vi "Z_State_heating.vi"(9 "Time":u32[](array[numeric])=[1000, 10000], 10 "Alarm":bool[](array[boolean])=[FALSE, FALSE], 11 "Z_In":T5={"Z_Source"=enum."local disabled", "Z_SetState"=enum."alarm", "ZM_State"=enum."initialization"}) -> (1 "t":u32, 3 "Z_Out":T4={"Z_Source"=enum."local disabled", "Z_State"=enum."alarm", "ZM_State"=enum."initialization"})   [LabVIEW 2019, in "Heating.lvlib"]
uses:
  Heating.lvlib
  ctl/Z_source.ctl
  ctl/Z_State.ctl
  ctl/ZM_State.ctl
  Trigers/RS.vi
  Timer Delay/Timer.vi
  Userlib.lvlib
panel:
  # "Alarm_L1"
  # "Alarm_L2"
  # "TsStop"
  # "T_check"
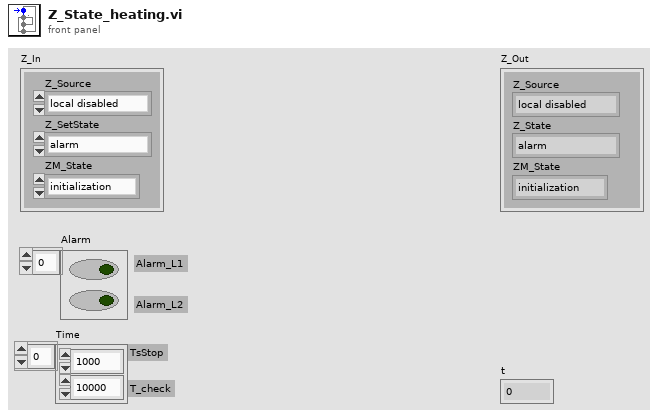
[diagram p1: front panel]
types:
  T1 = typedef "Heating.lvlib/Z_source.ctl" = enum8{"initialize", "local disabled", "local hand", "hand", "auto", "dist"}
  T2 = typedef "Heating.lvlib/Z_State.ctl" = enum8{"initialization", "alarm", "disabled", "not ready", "stop ready", "reserv", "switched off", "reserv2", "switched on", "check", "on min", "decrease out", "on", "increase out", "on max"}
  T3 = typedef "Heating.lvlib/ZM_State.ctl" = enum8{"initialization", "stop", "start_cmd", "contactor_on_cmd", "heating", "on", "stop_cmd", "power_down", "contactor_off_cmd", "cooling", "restart_delay"}
  T4 = cluster{"Z_Source":T1, "Z_State":T2, "ZM_State":T3}
  T5 = cluster{"Z_Source":T1, "Z_SetState":T2, "ZM_State":T3}
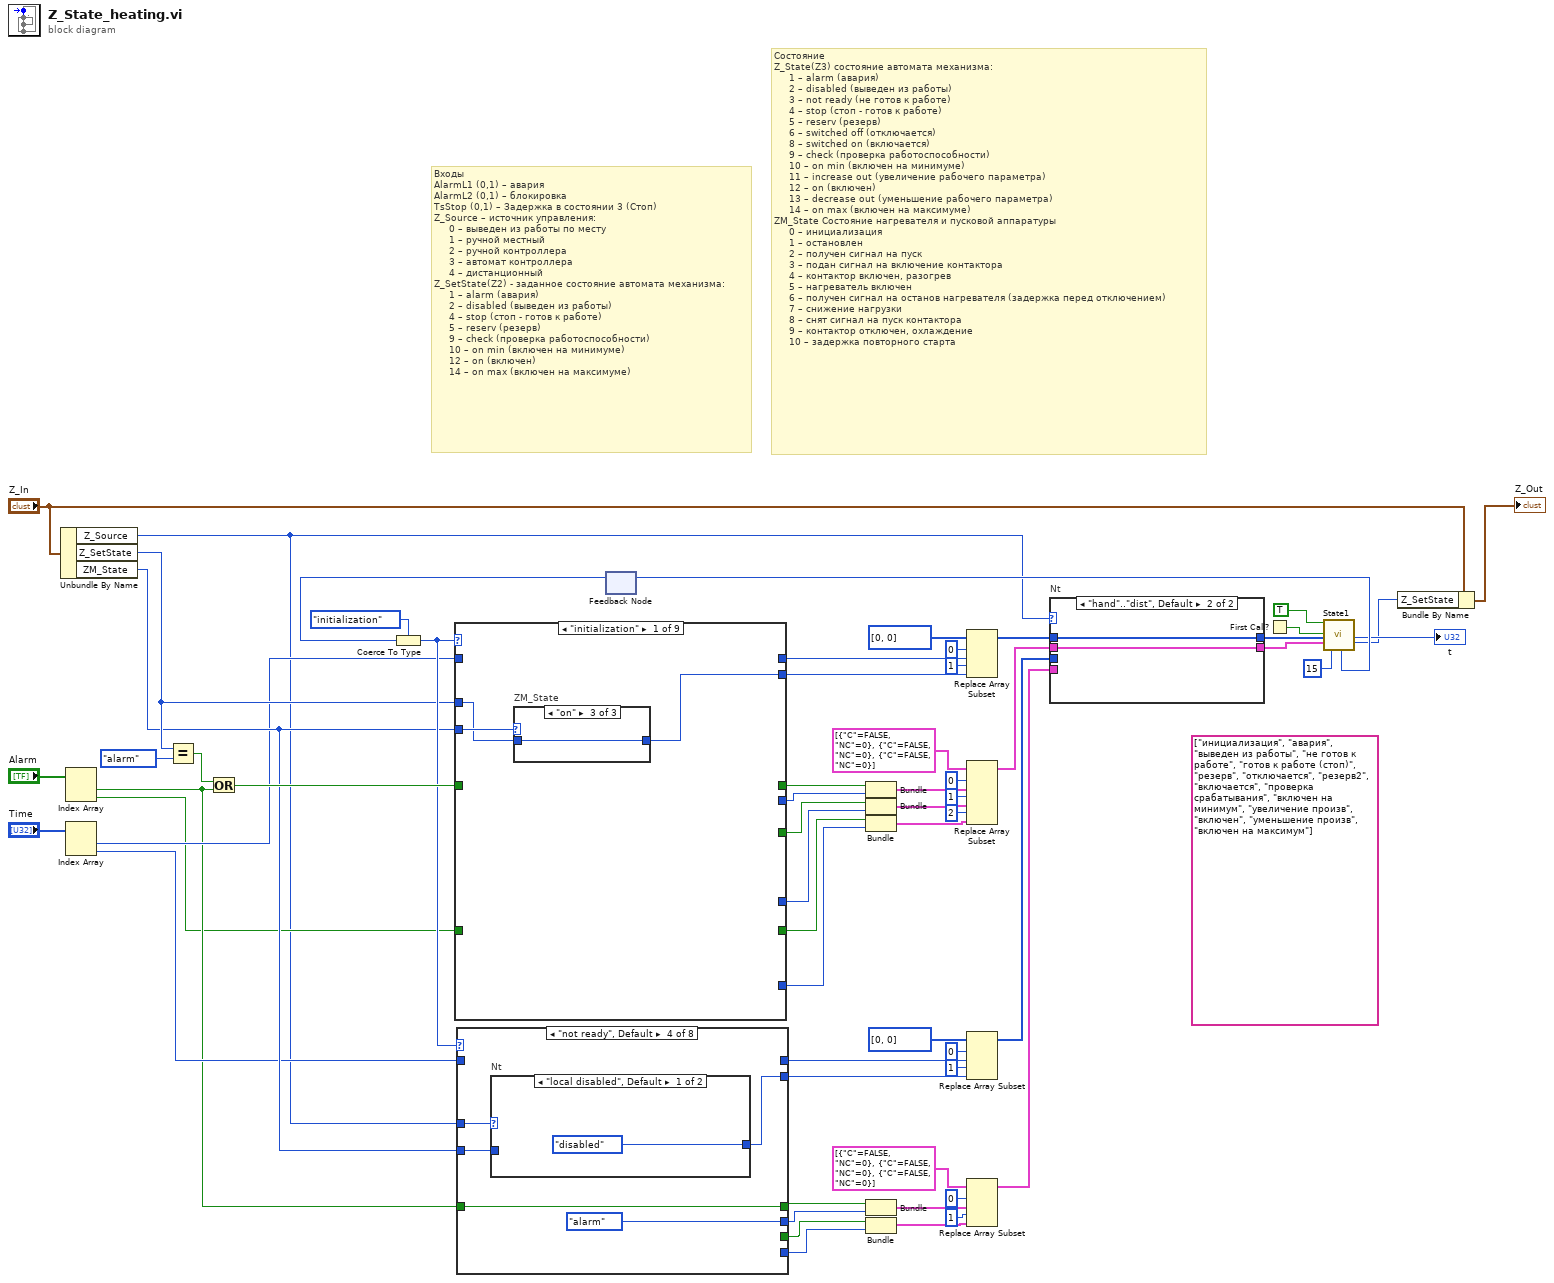
[diagram p0: block diagram]
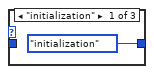
[diagram p3: hidden frame]
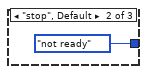
[diagram p4: hidden frame]
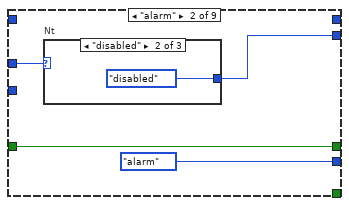
[diagram p5: hidden frame]
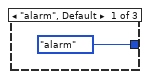
[diagram p6: hidden frame]
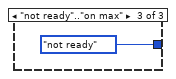
[diagram p7: hidden frame]
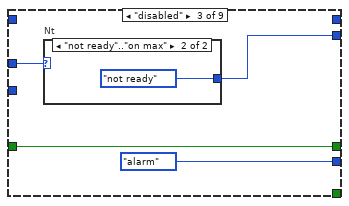
[diagram p8: hidden frame]
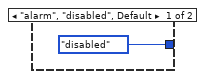
[diagram p9: hidden frame]
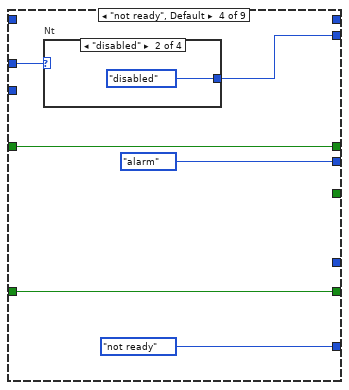
[diagram p10: hidden frame]
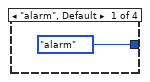
[diagram p11: hidden frame]
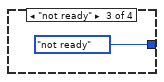
[diagram p12: hidden frame]
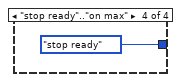
[diagram p13: hidden frame]
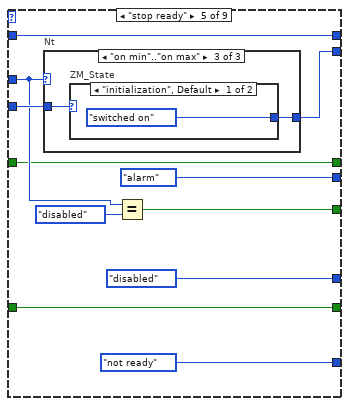
[diagram p14: hidden frame]
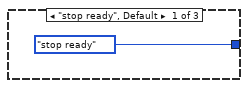
[diagram p15: hidden frame]
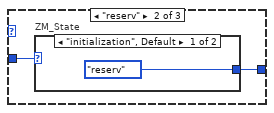
[diagram p16: hidden frame]
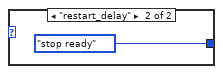
[diagram p17: hidden frame]
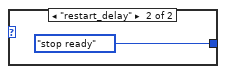
[diagram p18: hidden frame]
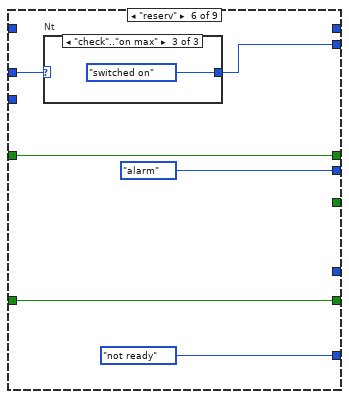
[diagram p19: hidden frame]
diagram:
  (unwired) string[] ["инициализация", "авария", "выведен из работы", "не готов к работе", "готов к работе (стоп)", "резерв", "отключается", "резерв2", "включается", "проверка срабатывания", "включен на минимум", "увеличение произв", "включен", "уменьшение произв", "включен на максимум"]
  # "Входы\nAlarmL1 (0,1) – авария\nAlarmL2 (0,1) – блокировка\nTsStop (0,1) – Задержка в состоянии 3 (Стоп)\nZ_Source – источник управления:\n     0 – выведен из работы по месту\n     1 – ручной местный\n     2 – ручной контроллера\n     3 – автомат контроллера\n     4 – дистанционный\nZ_SetState(Z2) - заданное состояние автомата механизма:\n     1 – alarm (авария)\n     2 – disabled (выведен из работы)\n     4 – stop (стоп - готов к работе)\n     5 – reserv (резерв)\n     9 – check (проверка работоспособности)\n     10 – on min (включен на минимуме)\n     12 – on (включен)\n     14 – on max (включен на максимуме)"
  # "Состояние\nZ_State(Z3) состояние автомата механизма:\n     1 – alarm (авария)\n     2 – disabled (выведен из работы)\n     3 – not ready (не готов к работе)\n     4 – stop (стоп - готов к работе)\n     5 – reserv (резерв)\n     6 – switched off (отключается)\n     8 – switched on (включается)\n     9 – check (проверка работоспособности)\n     10 – on min (включен на минимуме)\n     11 – increase out (увеличение рабочего параметра)\n     12 – on (включен)\n     13 – decrease out (уменьшение рабочего параметра)\n     14 – on max (включен на максимуме)\nZM_State Состояние нагревателя и пусковой аппаратуры\n     0 – инициализация\n     1 – остановлен\n     2 – получен сигнал на пуск\n     3 – подан сигнал на включение контактора\n     4 – контактор включен, разогрев\n     5 – нагреватель включен\n     6 – получен сигнал на останов нагревателя (задержка перед отключением)\n     7 – снижение нагрузки\n     8 – снят сигнал на пуск контактора\n     9 – контактор отключен, охлаждение\n     10 – задержка повторного старта"
  n1 = Unbundle By Name("Z_In") -> ("Z_Source"=w2:T1, "Z_SetState"=w55:T2, "ZM_State"=w54:T3)
  n2 = Index Array(array="Alarm") -> (element #1=w48:bool, element #2=w47:bool)  [unwired: 2 in]
  n3 = Index Array(array="Time") -> (element #1=w51:u32, element #2=w50:u32)  [unwired: 2 in]
  n4 = Equal?(x=w55, y=Z_State."alarm") -> (x = y?=w61:bool)
  n5 = Or(x=w61, y=w48) -> (x .or. y?=w60:bool)
  n6 = feedback #1() -> (w57:u32)  [unwired: 1 in]
  n7 = Coerce To Type(0:w57, 1:Z_State."initialization" ("Z_SetState")) -> (2:w56:T2)
  n8 = case shown="\"initialization\"" w56 {
    tunnel: w60 -> [_ w70 w77 w85 w95 w115 w127 w143 w158]
    tunnel: w55 -> [w62 w71 w78 w86 w99 w116 w128 w141 w154]
    tunnel: w47 -> [_ _ _ w83 w97 w114 w124 w144 w156]
    tunnel: w51 -> [_ _ _ _ w98 _ _ _ _]
    tunnel: w54 -> [w64 _ _ _ w100 _ w121 w147 _]
    tunnel: [_ _ _ Z_State."not ready" ("Z_SetState") Z_State."not ready" ("Z_SetState") Z_State."not ready" ("Z_SetState") w120 Z_State."switched off" ("Z_SetState") Z_State."switched off" ("Z_SetState")] -> w10
    tunnel: [_ _ _ _ w98 _ _ _ _] -> w16
    tunnel: [_ _ _ w83 w97 w114 w124 w146 w157] -> w9
    tunnel: [_ _ _ _ Z_State."disabled" ("Z_SetState") _ w125 _ _] -> w8
    tunnel: [_ _ _ _ w96 _ w126 _ _] -> w11
    tunnel: [_ Z_State."alarm" ("Z_SetState") Z_State."alarm" ("Z_SetState") Z_State."alarm" ("Z_SetState") Z_State."alarm" ("Z_SetState") Z_State."alarm" ("Z_SetState") Z_State."alarm" ("Z_SetState") Z_State."alarm" ("Z_SetState") Z_State."alarm" ("Z_SetState")] -> w12
    tunnel: [_ w70 w77 w85 w95 w115 w127 w143 w158] -> w13
    tunnel: [w63 w69 w76 w84 w94 w113 w123 w142 w154] -> w15
    frame "initialization" {
      n9 = case "ZM_State" shown="\"on\"" w64 {
        tunnel: [Z_State."initialization" ("Z_SetState") Z_State."not ready" ("Z_SetState") w67] -> w63
        tunnel: w62 -> [_ _ w67]
        frame "initialization" {
        }
        frame "stop", Default {
        }
        frame "on" {
        }
      }
    }
    frame "alarm" {
      n10 = case "Nt" shown="\"disabled\"" w71 {
        tunnel: [Z_State."alarm" ("Z_SetState") Z_State."disabled" ("Z_SetState") Z_State."not ready" ("Z_SetState")] -> w69
        frame "alarm", Default {
        }
        frame "disabled" {
        }
        frame "not ready".."on max" {
        }
      }
    }
    frame "disabled" {
      n11 = case "Nt" shown="\"not ready\"..\"on max\"" w78 {
        tunnel: [Z_State."disabled" ("Z_SetState") Z_State."not ready" ("Z_SetState")] -> w76
        frame "alarm", "disabled", Default {
        }
        frame "not ready".."on max" {
        }
      }
    }
    frame "not ready", Default {
      n12 = case "Nt" shown="\"disabled\"" w86 {
        tunnel: [Z_State."alarm" ("Z_SetState") Z_State."disabled" ("Z_SetState") Z_State."not ready" ("Z_SetState") Z_State."stop ready" ("Z_SetState")] -> w84
        frame "alarm", Default {
        }
        frame "disabled" {
        }
        frame "not ready" {
        }
        frame "stop ready".."on max" {
        }
      }
    }
    frame "stop ready" {
      n13 = case "Nt" shown="\"on min\"..\"on max\"" w99 {
        tunnel: [Z_State."stop ready" ("Z_SetState") w103 w107] -> w94
        tunnel: w100 -> [_ w104 w108]
        frame "stop ready", Default {
        }
        frame "reserv" {
          n14 = case "ZM_State" shown="\"initialization\", Default" w104 {
            tunnel: [Z_State."reserv" ("Z_SetState") Z_State."stop ready" ("Z_SetState")] -> w103
            frame "initialization", Default {
            }
            frame "restart_delay" {
            }
          }
        }
        frame "on min".."on max" {
          n15 = case "ZM_State" shown="\"initialization\", Default" w108 {
            tunnel: [Z_State."switched on" ("Z_SetState") Z_State."stop ready" ("Z_SetState")] -> w107
            frame "initialization", Default {
            }
            frame "restart_delay" {
            }
          }
        }
      }
      n16 = Equal?(x=w99, y=Z_State."disabled") -> (x = y?=w96:bool)
    }
    frame "reserv" {
      n17 = case "Nt" shown="\"check\"..\"on max\"" w116 {
        selector: w116 -> [w117 _ _]
        tunnel: [w117 Z_State."stop ready" ("Z_SetState") Z_State."switched on" ("Z_SetState")] -> w113
        frame "alarm".."not ready", "reserv" {
        }
        frame "stop ready", Default {
        }
        frame "check".."on max" {
        }
      }
    }
    frame "switched off" {
      n18 = case "Nt" shown="\"stop ready\", \"reserv\", \"check\", Default" w128 {
        tunnel: [w134 Z_State."switched on" ("Z_SetState")] -> w123
        tunnel: w121 -> [w135 _]
        frame "stop ready", "reserv", "check", Default {
          n19 = case "ZM_State" shown="\"initialization\", Default" w135 {
            tunnel: [Z_State."stop ready" ("Z_SetState") Z_State."switched off" ("Z_SetState")] -> w134
            frame "initialization", Default {
            }
            frame "stop_cmd".."cooling" {
            }
          }
        }
        frame "on min".."on max" {
        }
      }
      n20 = case "ZM_State" shown="\"stop_cmd\"..\"cooling\"" w121 {
        tunnel: [Z_State."disabled" ("Z_SetState") Z_State."switched off" ("Z_SetState")] -> w125
        frame "initialization", "stop", "restart_delay", Default {
        }
        frame "stop_cmd".."cooling" {
        }
      }
      n21 = case "ZM_State" shown="\"initialization\", \"stop\", \"restart_delay\", Default" w121 {
        tunnel: [Z_State."not ready" ("Z_SetState") Z_State."switched off" ("Z_SetState")] -> w120
        frame "initialization", "stop", "restart_delay", Default {
        }
        frame "stop_cmd".."cooling" {
        }
      }
      n22 = Equal?(x=w128, y=Z_State."disabled") -> (x = y?=w126:bool)
    }
    frame "switched on" {
      n23 = case "ZM_State" shown="\"on\"" w147 {
        tunnel: [Z_State."switched on" ("Z_SetState") w149] -> w142
        tunnel: w141 -> [_ w149]
        frame "initialization", Default {
        }
        frame "on" {
        }
      }
      n24 = case "Z2" shown="\"disabled\"..\"reserv\", Default" w141 {
        tunnel: [FALSE TRUE] -> w145
        frame "check".."on max" {
        }
        frame "disabled".."reserv", Default {
        }
      }
      n25 = Or(x=w145, y=w144) -> (x .or. y?=w146:bool)
    }
    frame "check".."on max" {
      n26 = case "Z2" shown="\"disabled\"..\"reserv\", Default" w154 {
        tunnel: [FALSE TRUE] -> w155
        frame "check".."on max" {
        }
        frame "disabled".."reserv", Default {
        }
      }
      n27 = Or(x=w155, y=w156) -> (x .or. y?=w157:bool)
    }
  }
  n28 = case shown="\"not ready\", Default" w56 {
    tunnel: w48 -> [_ w169 _ w180 w190 w200 w210 w220]
    tunnel: w2 -> [_ w168 w173 w179 w189 _ _ _]
    tunnel: w54 -> [w162 _ _ w177 w188 w199 w209 w218]
    tunnel: [_ _ _ _ _ _ w208 _] -> w3
    tunnel: [_ _ _ _ _ _ w207 _] -> w4
    tunnel: [_ Z_State."alarm" ("Z_SetState") _ Z_State."alarm" ("Z_SetState") Z_State."alarm" ("Z_SetState") Z_State."alarm" ("Z_SetState") Z_State."alarm" ("Z_SetState") Z_State."alarm" ("Z_SetState")] -> w5
    tunnel: [_ w169 _ w180 w190 w200 w210 w220] -> w6
    tunnel: [w161 w167 w172 w178 w187 w198 w208 w217] -> w7
    tunnel: w50 -> [_ _ _ _ _ _ w206 _]
    tunnel: [_ _ _ _ _ _ w206 _] -> w14
    frame "initialization" {
      n29 = case "ZM_State" shown="\"on\"" w162 {
        tunnel: [Z_State."initialization" ("Z_SetState") Z_State."not ready" ("Z_SetState") Z_State."check" ("Z_SetState")] -> w161
        frame "initialization" {
        }
        frame "stop", Default {
        }
        frame "on" {
        }
      }
    }
    frame "alarm" {
      n30 = case "Nt" shown="\"local disabled\", Default" w168 {
        tunnel: [Z_State."disabled" ("Z_SetState") Z_State."not ready" ("Z_SetState")] -> w167
        frame "local disabled", Default {
        }
        frame "local hand" {
        }
      }
    }
    frame "disabled", "stop ready", "reserv", "reserv2" {
      n31 = case "Nt" shown="\"local disabled\", Default" w173 {
        tunnel: [Z_State."disabled" ("Z_SetState") Z_State."not ready" ("Z_SetState")] -> w172
        frame "local disabled", Default {
        }
        frame "local hand" {
        }
      }
    }
    frame "not ready", Default {
      n32 = case "Nt" shown="\"local disabled\", Default" w179 {
        tunnel: [Z_State."disabled" ("Z_SetState") w183] -> w178
        tunnel: w177 -> [_ w182]
        frame "local disabled", Default {
        }
        frame "local hand" {
          n33 = case "ZM_State" shown="\"contactor_on_cmd\"..\"on\"" w182 {
            tunnel: [Z_State."not ready" ("Z_SetState") Z_State."switched on" ("Z_SetState")] -> w183
            frame "initialization", Default {
            }
            frame "contactor_on_cmd".."on" {
            }
          }
        }
      }
    }
    frame "switched off" {
      n34 = case "Nt" shown="\"local hand\", Default" w189 {
        tunnel: [Z_State."disabled" ("Z_SetState") w192] -> w187
        tunnel: w188 -> [_ w193]
        frame "local disabled" {
        }
        frame "local hand", Default {
          n35 = case "ZM_State" shown="\"contactor_on_cmd\"..\"on\"" w193 {
            tunnel: [Z_State."not ready" ("Z_SetState") Z_State."switched on" ("Z_SetState") Z_State."switched off" ("Z_SetState")] -> w192
            frame "initialization".."start_cmd", "restart_delay", Default {
            }
            frame "contactor_on_cmd".."on" {
            }
            frame "stop_cmd".."cooling" {
            }
          }
        }
      }
    }
    frame "switched on" {
      n36 = case "Nt" shown="\"stop_cmd\"..\"cooling\"" w199 {
        tunnel: [Z_State."not ready" ("Z_SetState") Z_State."switched on" ("Z_SetState") Z_State."check" ("Z_SetState") Z_State."switched off" ("Z_SetState")] -> w198
        frame "initialization", "stop", "restart_delay", Default {
        }
        frame "start_cmd".."heating" {
        }
        frame "on" {
        }
        frame "stop_cmd".."cooling" {
        }
      }
    }
    frame "check" {
      n37 = case "ZM_State" shown="\"initialization\"..\"start_cmd\", Default" w209 {
        tunnel: [Z_State."not ready" ("Z_SetState") Z_State."on" ("Z_SetState") Z_State."switched off" ("Z_SetState")] -> w208
        tunnel: [TRUE FALSE TRUE] -> w207
        frame "initialization".."start_cmd", Default {
        }
        frame "contactor_on_cmd".."power_down" {
        }
        frame "contactor_off_cmd".."restart_delay" {
        }
      }
    }
    frame "on min".."on max" {
      n38 = case "ZM_State" shown="\"contactor_off_cmd\"..\"restart_delay\"" w218 {
        tunnel: [Z_State."not ready" ("Z_SetState") Z_State."on" ("Z_SetState") Z_State."switched off" ("Z_SetState")] -> w217
        frame "initialization".."start_cmd", Default {
        }
        frame "contactor_on_cmd".."power_down" {
        }
        frame "contactor_off_cmd".."restart_delay" {
        }
      }
    }
  }
  n39 = Bundle(w13, "Z_SetState"=w12) -> (w38:cluster{bool, "Z_SetState":T2})  [unwired: 1 in]
  n40 = Bundle(w11, "Z_SetState"=w8) -> (w35:cluster{bool, "Z_SetState":T2})  [unwired: 1 in]
  n41 = Bundle("Alarm"=w9, "Z_SetState"=w10) -> (w34:cluster{"Alarm":bool, "Z_SetState":T2})  [unwired: 1 in]
  n42 = Bundle("Alarm"=w6, "Z_SetState"=w5) -> (w31:cluster{"Alarm":bool, "Z_SetState":T2})  [unwired: 1 in]
  n43 = Bundle(w4, "Z_SetState"=w3) -> (w33:cluster{bool, "Z_SetState":T2})  [unwired: 1 in]
  n44 = Replace Array Subset(array=u32[] [0, 0] ("appended array"), new element #1=w16, index #1=0 ("index"), new element #2=w15, index #2=1 ("index")) -> (w23:u32[])
  n45 = Replace Array Subset(array=cluster{"C":bool, "NC":u32}[] [{"C"=FALSE, "NC"=0}, {"C"=FALSE, "NC"=0}, {"C"=FALSE, "NC"=0}] ("appended array"), new element #1=w38, index #1=0 ("index"), new element #2=w35, index #2=1 ("index"), new element #3=w34, index #3=2 ("index")) -> (w21:cluster{"C":bool, "NC":u32}[])
  n46 = Replace Array Subset(array=u32[] [0, 0] ("appended array"), new element #1=w14, index #1=0 ("index"), new element #2=w7, index #2=1 ("index")) -> (w25:u32[])
  n47 = Replace Array Subset(array=cluster{"C":bool, "NC":u32}[] [{"C"=FALSE, "NC"=0}, {"C"=FALSE, "NC"=0}, {"C"=FALSE, "NC"=0}] ("appended array"), new element #1=w31, index #1=0 ("index"), new element #2=w33, index #2=1 ("index")) -> (w24:cluster{"C":bool, "NC":u32}[])
  n48 = case "Nt" shown="\"hand\"..\"dist\", Default" w2 {
    tunnel: w23 -> [_ w227]
    tunnel: w21 -> [_ w226]
    tunnel: [w224 w227] -> w22
    tunnel: [w225 w226] -> w20
    tunnel: w25 -> [w224 _]
    tunnel: w24 -> [w225 _]
    frame "local disabled", "local hand" {
    }
    frame "hand".."dist", Default {
    }
  }
  n49 = First Call?() -> (First Call?: T/F=w45:bool)
  n50 = call "State1.vi"("Start"=TRUE, "Reset"=w45, "T_table"=w22, "C_table"=w20, "End step"=u32 15) -> ("N next"=w19:u32, "t"=→"t":u32, "N curr"=w17:u32)  [unwired: 9 in, 3 out]
  n51 = feedback-in #1(w19) -> ()
  n52 = Bundle By Name(cluster="Z_In", "Z_SetState"=w17) -> (→"Z_Out":T5)
